vi "Module time text to numbers.vi"(1 "Module List Text":T2(array[cluster])=[{"Enable"=TRUE, "Abs Start Time"=" 900.000", "Module"=1, "String"="kill Rb MOT", "Array"=["b", "0"]}, {"Enable"=TRUE, "Abs Start Time"="   1.000", "Module"=0, "String"="dynamic DAC trigger", "Array"=["D", "14"]}, {"Enable"=TRUE, "Abs Start Time"="  21.000", "Module"=1, "String"="trigger down", "Array"=["D", "14"]}, {"Enable"=TRUE, "Abs Start Time"=" 947.000", "Module"=19, "String"="", "Array"=[]}, {"Enable"=TRUE, "Abs Start Time"=" 945.000", "Module"=20, "String"="K trap freq for CMOT", "Array"=["5", "4.6"]}, {"Enable"=TRUE, "Abs Start Time"=" 945.000", "Module"=20, "String"="E/W shim for Qtrap loading", "Array"=["0", "-1"]}, {"Enable"=TRUE, "Abs Start Time"=" 945.000", "Module"=20, "String"="U/D shim for Qtrap loading", "Array"=["1", "-1"]}, {"Enable"=TRUE, "Abs Start Time"=" 945.000", "Module"=20, "String"="N/S shim for Qtrap loading", "Array"=["2", "2"]}, {"Enable"=TRUE, "Abs Start Time"=" 997.000", "Module"=20, "String"="repump K freq for OP", "Array"=["3", "0.05"]}, {"Enable"=TRUE, "Abs Start Time"=" 994.500", "Module"=20, "String"="E/W shim for molasses 0", "Array"=["0", "-1"]}, {"Enable"=TRUE, "Abs Start Time"=" 994.500", "Module"=20, "String"="U/D shim for molasses -0.6", "Array"=["1", "0.1"]}, {"Enable"=TRUE, "Abs Start Time"=" 994.500", "Module"=20, "String"="N/S shim for molasses 0", "Array"=["2", "2"]}, {"Enable"=TRUE, "Abs Start Time"=" 995.500", "Module"=8, "String"="", "Array"=["", ""]}, {"Enable"=TRUE, "Abs Start Time"=" 997.100", "Module"=1, "String"="close Rb shutter(takes 1.4 ms", "Array"=["B", "0"]}, {"Enable"=TRUE, "Abs Start Time"=" 998.500", "Module"=12, "String"="\n", "Array"=[]}, {"Enable"=FALSE, "Abs Start Time"=" 998.500", "Module"=0, "String"="scope trigger", "Array"=["c", "7"]}, {"Enable"=FALSE, "Abs Start Time"=" 999.000", "Module"=1, "String"="", "Array"=["c", "7"]}, {"Enable"=TRUE, "Abs Start Time"="1000.000", "Module"=14, "String"="", "Array"=[]}, {"Enable"=TRUE, "Abs Start Time"="1000.000", "Module"=20, "String"="K trap freq for MOT", "Array"=["5", "4.3"]}, {"Enable"=TRUE, "Abs Start Time"="1000.000", "Module"=20, "String"=" K repump freq for MOT freq", "Array"=["3", "0"]}, {"Enable"=TRUE, "Abs Start Time"="1000.000", "Module"=20, "String"="E/W shim for Qtrap", "Array"=["0", "0"]}, {"Enable"=TRUE, "Abs Start Time"="1000.000", "Module"=20, "String"="U/D shim for Qtrap", "Array"=["1", "0"]}, {"Enable"=TRUE, "Abs Start Time"="1000.000", "Module"=20, "String"="N/S shim for Qtrap", "Array"=["2", "0"]}, {"Enable"=TRUE, "Abs Start Time"="1000.000", "Module"=20, "String"="U/D cart shim on", "Array"=["4", "8"]}, {"Enable"=FALSE, "Abs Start Time"="1000.000", "Module"=10, "String"="", "Array"=["2400"]}, {"Enable"=FALSE, "Abs Start Time"="1000.000", "Module"=0, "String"="laser unlock", "Array"=["A", "1"]}] {"Module" items=["TTL high                                                                                 ", "TTL low                          ", "Camera Strobe                   ", "Defaults                           ", "Fluorescence pulse           ", "IP trap                         ", "Kinetics OD image          ", "MOT light only                ", "MOT off                                   ", "MOT on                         ", "Move cart                      ", "OD image                     ", "Optical pumping          ", "Picture                             ", "Quadrupole trap             ", "Utility Module 01          ", "Utility Module 02           ", "Utility Module 03           ", "Utility Module 04           ", "CMOT", "Static DAQ"]}) -> (0 "Module List Numbers":T1(array[cluster])=[{"Enable"=TRUE, "Abs Start Time"=900.0, "Module"=1, "String"="kill Rb MOT", "Array"=["b", "0"]}, {"Enable"=TRUE, "Abs Start Time"=1.0, "Module"=0, "String"="dynamic DAC trigger", "Array"=["D", "14"]}, {"Enable"=TRUE, "Abs Start Time"=21.0, "Module"=1, "String"="trigger down", "Array"=["D", "14"]}, {"Enable"=TRUE, "Abs Start Time"=947.0, "Module"=19, "String"="", "Array"=[]}, {"Enable"=TRUE, "Abs Start Time"=945.0, "Module"=20, "String"="K trap freq for CMOT", "Array"=["5", "4.6"]}, {"Enable"=TRUE, "Abs Start Time"=945.0, "Module"=20, "String"="E/W shim for Qtrap loading", "Array"=["0", "-1"]}, {"Enable"=TRUE, "Abs Start Time"=945.0, "Module"=20, "String"="U/D shim for Qtrap loading", "Array"=["1", "-1"]}, {"Enable"=TRUE, "Abs Start Time"=945.0, "Module"=20, "String"="N/S shim for Qtrap loading", "Array"=["2", "2"]}, {"Enable"=TRUE, "Abs Start Time"=997.0, "Module"=20, "String"="repump K freq for OP", "Array"=["3", "0.05"]}, {"Enable"=TRUE, "Abs Start Time"=994.5, "Module"=20, "String"="E/W shim for molasses 0", "Array"=["0", "-1"]}, {"Enable"=TRUE, "Abs Start Time"=994.5, "Module"=20, "String"="U/D shim for molasses -0.6", "Array"=["1", "0.1"]}, {"Enable"=TRUE, "Abs Start Time"=994.5, "Module"=20, "String"="N/S shim for molasses 0", "Array"=["2", "2"]}, {"Enable"=TRUE, "Abs Start Time"=995.5, "Module"=8, "String"="", "Array"=["", ""]}, {"Enable"=TRUE, "Abs Start Time"=997.1, "Module"=1, "String"="close Rb shutter(takes 1.4 ms", "Array"=["B", "0"]}, {"Enable"=TRUE, "Abs Start Time"=998.5, "Module"=12, "String"="\n", "Array"=[]}, {"Enable"=FALSE, "Abs Start Time"=998.5, "Module"=0, "String"="scope trigger", "Array"=["c", "7"]}, {"Enable"=FALSE, "Abs Start Time"=999.0, "Module"=1, "String"="", "Array"=["c", "7"]}, {"Enable"=TRUE, "Abs Start Time"=1000.0, "Module"=14, "String"="", "Array"=[]}, {"Enable"=TRUE, "Abs Start Time"=1000.0, "Module"=20, "String"="K trap freq for MOT", "Array"=["5", "4.3"]}, {"Enable"=TRUE, "Abs Start Time"=1000.0, "Module"=20, "String"=" K repump freq for MOT freq", "Array"=["3", "0"]}, {"Enable"=TRUE, "Abs Start Time"=1000.0, "Module"=20, "String"="E/W shim for Qtrap", "Array"=["0", "0"]}, {"Enable"=TRUE, "Abs Start Time"=1000.0, "Module"=20, "String"="U/D shim for Qtrap", "Array"=["1", "0"]}, {"Enable"=TRUE, "Abs Start Time"=1000.0, "Module"=20, "String"="N/S shim for Qtrap", "Array"=["2", "0"]}, {"Enable"=TRUE, "Abs Start Time"=1000.0, "Module"=20, "String"="U/D cart shim on", "Array"=["4", "8"]}, {"Enable"=FALSE, "Abs Start Time"=1000.0, "Module"=10, "String"="", "Array"=["2400"]}, {"Enable"=FALSE, "Abs Start Time"=1000.0, "Module"=0, "String"="laser unlock", "Array"=["A", "1"]}, {"Enable"=FALSE, "Abs Start Time"=4000.0, "Module"=1, "String"="", "Array"=["A", "12"]}] {"Module" items=["TTL high                                                                                 ", "TTL low                          ", "Camera Strobe                   ", "Defaults                           ", "Fluorescence pulse           ", "IP trap                         ", "Kinetics OD image          ", "MOT light only                ", "MOT off                                   ", "MOT on                         ", "Move cart                      ", "OD image                     ", "Optical pumping          ", "Picture                             ", "Quadrupole trap             ", "Utility Module 01          ", "Utility Module 02           ", "Utility Module 03           ", "Utility Module 04           ", "CMOT", "Static DAQ"]; "Abs Start Time" format="%.3f"})   [LabVIEW 2017]
doc: "This vi converts the format of a single module list, converting the times from text to numbers."
panel:
  in  "Empty Module List Numbers":T1(array[cluster])=[{"Enable"=TRUE, "Abs Start Time"=900.0, "Module"=1, "String"="kill Rb MOT", "Array"=["b", "0"]}, {"Enable"=TRUE, "Abs Start Time"=1.0, "Module"=0, "String"="dynamic DAC trigger", "Array"=["D", "14"]}, {"Enable"=TRUE, "Abs Start Time"=21.0, "Module"=1, "String"="trigger down", "Array"=["D", "14"]}, {"Enable"=TRUE, "Abs Start Time"=947.0, "Module"=19, "String"="", "Array"=[]}, {"Enable"=TRUE, "Abs Start Time"=945.0, "Module"=20, "String"="K trap freq for CMOT", "Array"=["5", "4.6"]}, {"Enable"=TRUE, "Abs Start Time"=945.0, "Module"=20, "String"="E/W shim for Qtrap loading", "Array"=["0", "-1"]}, {"Enable"=TRUE, "Abs Start Time"=945.0, "Module"=20, "String"="U/D shim for Qtrap loading", "Array"=["1", "-1"]}, {"Enable"=TRUE, "Abs Start Time"=945.0, "Module"=20, "String"="N/S shim for Qtrap loading", "Array"=["2", "2"]}, {"Enable"=TRUE, "Abs Start Time"=997.0, "Module"=20, "String"="repump K freq for OP", "Array"=["3", "0.05"]}, {"Enable"=TRUE, "Abs Start Time"=994.5, "Module"=20, "String"="E/W shim for molasses 0", "Array"=["0", "-1"]}, {"Enable"=TRUE, "Abs Start Time"=994.5, "Module"=20, "String"="U/D shim for molasses -0.6", "Array"=["1", "0.1"]}, {"Enable"=TRUE, "Abs Start Time"=994.5, "Module"=20, "String"="N/S shim for molasses 0", "Array"=["2", "2"]}, {"Enable"=TRUE, "Abs Start Time"=995.5, "Module"=8, "String"="", "Array"=["", ""]}, {"Enable"=TRUE, "Abs Start Time"=997.1, "Module"=1, "String"="close Rb shutter(takes 1.4 ms", "Array"=["B", "0"]}, {"Enable"=TRUE, "Abs Start Time"=998.5, "Module"=12, "String"="\n", "Array"=[]}, {"Enable"=FALSE, "Abs Start Time"=998.5, "Module"=0, "String"="scope trigger", "Array"=["c", "7"]}, {"Enable"=FALSE, "Abs Start Time"=999.0, "Module"=1, "String"="", "Array"=["c", "7"]}, {"Enable"=TRUE, "Abs Start Time"=1000.0, "Module"=14, "String"="", "Array"=[]}, {"Enable"=TRUE, "Abs Start Time"=1000.0, "Module"=20, "String"="K trap freq for MOT", "Array"=["5", "4.3"]}, {"Enable"=TRUE, "Abs Start Time"=1000.0, "Module"=20, "String"=" K repump freq for MOT freq", "Array"=["3", "0"]}, {"Enable"=TRUE, "Abs Start Time"=1000.0, "Module"=20, "String"="E/W shim for Qtrap", "Array"=["0", "0"]}, {"Enable"=TRUE, "Abs Start Time"=1000.0, "Module"=20, "String"="U/D shim for Qtrap", "Array"=["1", "0"]}, {"Enable"=TRUE, "Abs Start Time"=1000.0, "Module"=20, "String"="N/S shim for Qtrap", "Array"=["2", "0"]}, {"Enable"=TRUE, "Abs Start Time"=1000.0, "Module"=20, "String"="U/D cart shim on", "Array"=["4", "8"]}, {"Enable"=FALSE, "Abs Start Time"=1000.0, "Module"=10, "String"="", "Array"=["2400"]}, {"Enable"=FALSE, "Abs Start Time"=1000.0, "Module"=0, "String"="laser unlock", "Array"=["A", "1"]}, {"Enable"=FALSE, "Abs Start Time"=4000.0, "Module"=1, "String"="", "Array"=["A", "12"]}, {"Enable"=FALSE, "Abs Start Time"=0.0, "Module"=0, "String"="", "Array"=[]}, {"Enable"=FALSE, "Abs Start Time"=0.0, "Module"=0, "String"="", "Array"=[]}, {"Enable"=FALSE, "Abs Start Time"=0.0, "Module"=0, "String"="", "Array"=[]}, {"Enable"=FALSE, "Abs Start Time"=0.0, "Module"=0, "String"="", "Array"=[]}, {"Enable"=FALSE, "Abs Start Time"=0.0, "Module"=0, "String"="", "Array"=[]}, {"Enable"=FALSE, "Abs Start Time"=0.0, "Module"=0, "String"="", "Array"=[]}, {"Enable"=FALSE, "Abs Start Time"=0.0, "Module"=0, "String"="", "Array"=[]}, {"Enable"=FALSE, "Abs Start Time"=0.0, "Module"=0, "String"="", "Array"=[]}, {"Enable"=FALSE, "Abs Start Time"=0.0, "Module"=0, "String"="", "Array"=[]}, {"Enable"=FALSE, "Abs Start Time"=0.0, "Module"=0, "String"="", "Array"=[]}, {"Enable"=FALSE, "Abs Start Time"=0.0, "Module"=0, "String"="", "Array"=[]}, {"Enable"=FALSE, "Abs Start Time"=0.0, "Module"=0, "String"="", "Array"=[]}, {"Enable"=FALSE, "Abs Start Time"=0.0, "Module"=0, "String"="", "Array"=[]}, {"Enable"=FALSE, "Abs Start Time"=0.0, "Module"=0, "String"="", "Array"=[]}, {"Enable"=FALSE, "Abs Start Time"=0.0, "Module"=0, "String"="", "Array"=[]}, {"Enable"=FALSE, "Abs Start Time"=0.0, "Module"=0, "String"="", "Array"=[]}, {"Enable"=FALSE, "Abs Start Time"=0.0, "Module"=0, "String"="", "Array"=[]}, {"Enable"=FALSE, "Abs Start Time"=0.0, "Module"=0, "String"="", "Array"=[]}, {"Enable"=FALSE, "Abs Start Time"=0.0, "Module"=0, "String"="", "Array"=[]}, {"Enable"=FALSE, "Abs Start Time"=0.0, "Module"=0, "String"="", "Array"=[]}, {"Enable"=FALSE, "Abs Start Time"=0.0, "Module"=0, "String"="", "Array"=[]}, {"Enable"=FALSE, "Abs Start Time"=0.0, "Module"=0, "String"="", "Array"=[]}, {"Enable"=FALSE, "Abs Start Time"=0.0, "Module"=0, "String"="", "Array"=[]}, {"Enable"=FALSE, "Abs Start Time"=0.0, "Module"=0, "String"="", "Array"=[]}, {"Enable"=FALSE, "Abs Start Time"=0.0, "Module"=0, "String"="", "Array"=[]}, {"Enable"=FALSE, "Abs Start Time"=0.0, "Module"=0, "String"="", "Array"=[]}, {"Enable"=FALSE, "Abs Start Time"=0.0, "Module"=0, "String"="", "Array"=[]}, {"Enable"=FALSE, "Abs Start Time"=0.0, "Module"=0, "String"="", "Array"=[]}, {"Enable"=FALSE, "Abs Start Time"=0.0, "Module"=0, "String"="", "Array"=[]}, {"Enable"=FALSE, "Abs Start Time"=0.0, "Module"=0, "String"="", "Array"=[]}, {"Enable"=FALSE, "Abs Start Time"=0.0, "Module"=0, "String"="", "Array"=[]}, {"Enable"=FALSE, "Abs Start Time"=0.0, "Module"=0, "String"="", "Array"=[]}, {"Enable"=TRUE, "Abs Start Time"=0.0, "Module"=0, "String"="", "Array"=[]}, {"Enable"=FALSE, "Abs Start Time"=0.0, "Module"=0, "String"="", "Array"=[]}, {"Enable"=FALSE, "Abs Start Time"=0.0, "Module"=0, "String"="", "Array"=[]}, {"Enable"=FALSE, "Abs Start Time"=0.0, "Module"=0, "String"="", "Array"=[]}, {"Enable"=FALSE, "Abs Start Time"=0.0, "Module"=0, "String"="", "Array"=[]}, {"Enable"=FALSE, "Abs Start Time"=0.0, "Module"=0, "String"="", "Array"=[]}, {"Enable"=FALSE, "Abs Start Time"=0.0, "Module"=0, "String"="", "Array"=[]}, {"Enable"=FALSE, "Abs Start Time"=0.0, "Module"=0, "String"="", "Array"=[]}, {"Enable"=FALSE, "Abs Start Time"=0.0, "Module"=0, "String"="", "Array"=[]}, {"Enable"=FALSE, "Abs Start Time"=0.0, "Module"=0, "String"="", "Array"=[]}, {"Enable"=FALSE, "Abs Start Time"=0.0, "Module"=0, "String"="", "Array"=[]}, {"Enable"=FALSE, "Abs Start Time"=0.0, "Module"=0, "String"="", "Array"=[]}, {"Enable"=FALSE, "Abs Start Time"=0.0, "Module"=0, "String"="", "Array"=[]}, {"Enable"=FALSE, "Abs Start Time"=0.0, "Module"=0, "String"="", "Array"=[]}, {"Enable"=FALSE, "Abs Start Time"=0.0, "Module"=0, "String"="", "Array"=[]}, {"Enable"=FALSE, "Abs Start Time"=0.0, "Module"=0, "String"="", "Array"=[]}, {"Enable"=FALSE, "Abs Start Time"=0.0, "Module"=0, "String"="", "Array"=[]}, {"Enable"=FALSE, "Abs Start Time"=0.0, "Module"=0, "String"="", "Array"=[]}, {"Enable"=FALSE, "Abs Start Time"=0.0, "Module"=0, "String"="", "Array"=[]}, {"Enable"=FALSE, "Abs Start Time"=0.0, "Module"=0, "String"="", "Array"=[]}, {"Enable"=TRUE, "Abs Start Time"=0.0, "Module"=0, "String"="", "Array"=[]}] {"Module" items=["TTL high                                                                                 ", "TTL low                          ", "Camera Strobe                   ", "Defaults                           ", "Fluorescence pulse           ", "IP trap                         ", "Kinetics OD image          ", "MOT light only                ", "MOT off                                   ", "MOT on                         ", "Move cart                      ", "OD image                     ", "Optical pumping          ", "Picture                             ", "Quadrupole trap             ", "Utility Module 01          ", "Utility Module 02           ", "Utility Module 03           ", "Utility Module 04           ", "CMOT", "Static DAQ"]; "Abs Start Time" format="%.3f"}
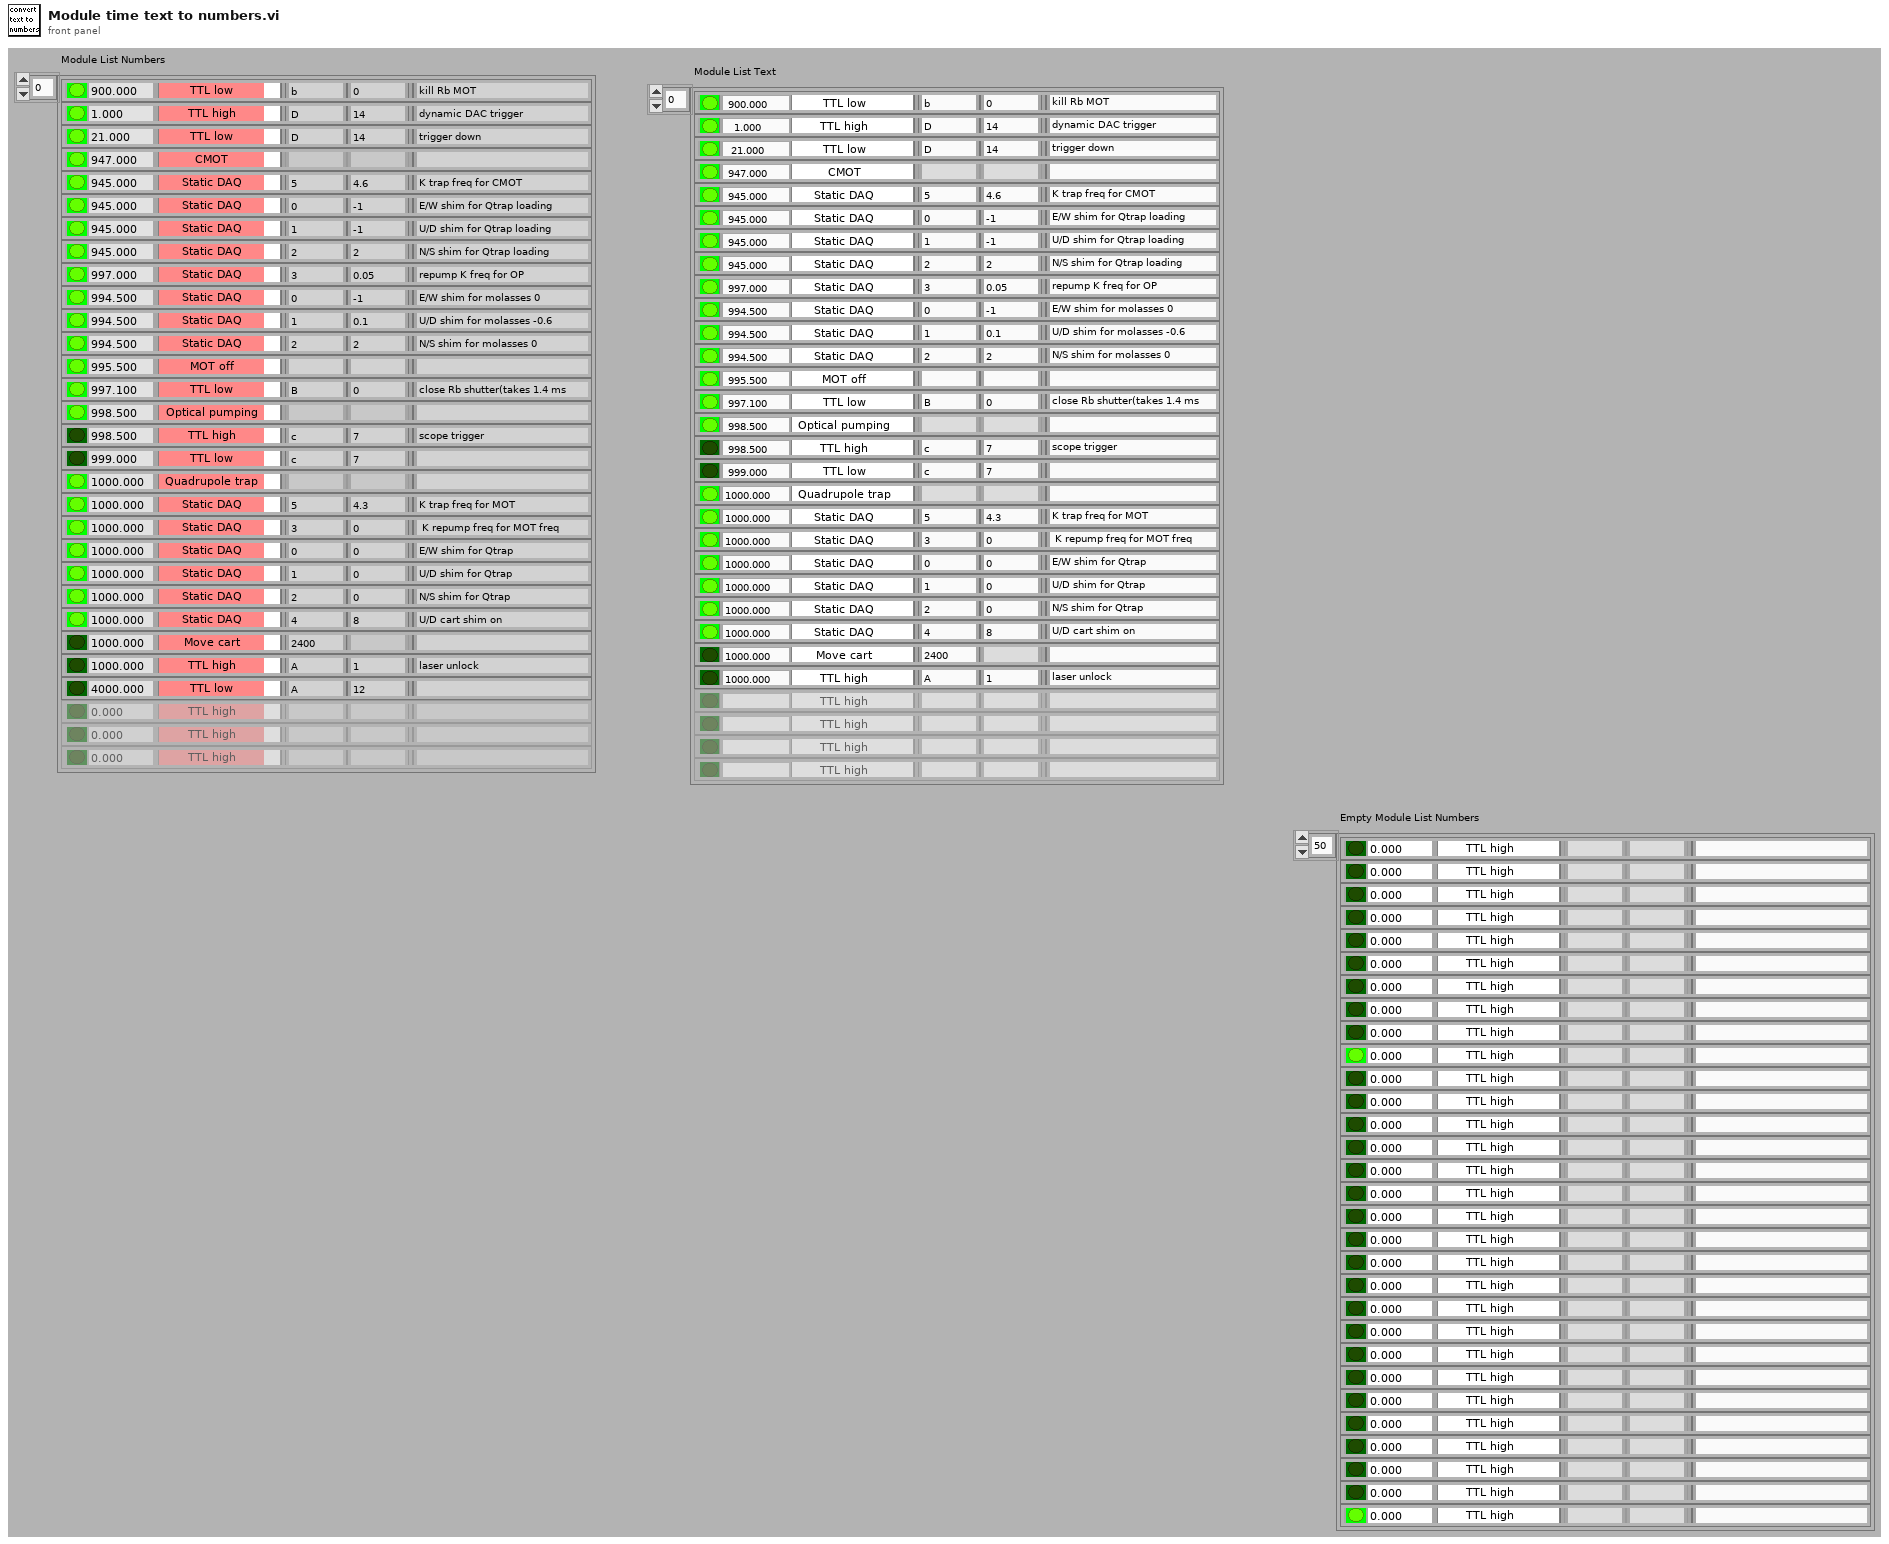
[diagram p1: front panel]
types:
  T1 = cluster{"Enable":bool, "Abs Start Time":dbl, "Module":u16, "String":string, "Array":string[]}[]
  T2 = cluster{"Enable":bool, "Abs Start Time":string, "Module":u16, "String":string, "Array":string[]}[]
  T3 = cluster{"Enable":bool, "Abs Start Time":dbl, "Module":u16, "String":string, "Array":string[]}
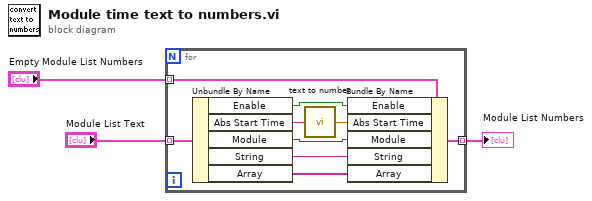
[diagram p0: block diagram]
diagram:
  n1 = for {
    tunnel: "Module List Text" -> [w8] mode=indexing
    tunnel: "Empty Module List Numbers" -> [w7] mode=indexing
    tunnel: [w6] -> w1 mode=indexing
    n2 = Unbundle By Name(w8) -> ("Enable"=w9:bool, "Abs Start Time"=w5:string, "Module"=w12:u16, "String"=w11:string, "Array"=w10:string[])
    n3 = call "text to number.vi"("text"=w5) -> ("number"=w4:dbl)
    n4 = Bundle By Name(cluster=w7, "Enable"=w9, "Abs Start Time"=w4, "Module"=w12, "String"=w11, "Array"=w10) -> (w6:T3)
  }
  "Module List Numbers" <- w1
